vi "Mapping v10.5.2.vi"(5 "Simulate Spectra":bool, 7 "Simulate Drive":bool) -> ()   [LabVIEW 2010]
uses:
  ESA-C/TypeDefs/ESA-C Connection Settings.ctl
  TypeDefs/Mapping Spectra Params.ctl
  TypeDefs/Mapping Drive Params.ctl
  ESA-C/TypeDefs/ESA-C Set Positions.ctl
  ESA-C/TypeDefs/ESA-C Current Values.ctl
  iHR550/TypeDefs/iHR Current Values.ctl
  ITC503/TypeDefs/ITC503 Current Values.ctl
  TypeDefs/Mapping Input Parameters v10.5.1.ctl
  Symphony/TypeDefs/Symphony Area Format.ctl
  <vilib>/Utility/miscctls.llb/LVPointTypeDef.ctl
  Global Variables.vi
panel:
  in  "Input Parameters":T1={"Drive Connection Settings"={"Objective GPIB-Port"=4, "Stage GPIB-Port"=4, "Drive Selector"=0, "Drive Velocity (V/s)"=5.0}, "ITC503 Current Values"={"ITC503 Heater"=0.0, "ITC503 Temperature"=0.0, "ITC503 P"=0.0, "ITC503 I"=0.0, "ITC503 D"=0.0, "ITC503 Setpoint"=0.0, "ITC503 Gradient"=0.0, "ITC503 Heater Auto"=FALSE, "ITC503 PID Auto"=FALSE}, "Wavelengths (nm)"=[], "Drive Current Values"={"Voltages"={"Drive X Voltage"=0.0, "Drive Y Voltage"=0.0, "Drive Z Voltage"=0.0}, "Position"={"Drive X Position"=0.0, "Drive Y Position"=0.0, "Drive Z Position"=0.0}}, "iHR Current Values"={"iHR 550 Front Entrance"=0.0, "iHR550 Side Exit"=0.0, "iHR550 Wavelength"=897.9988, "iHR550 Exit Mirror"=2, "iHR550 Grating"="1", "Grating Index"=1}, "Spectra Settings"={"Integration Time"=1.0, "Repetitions"=1, "Mapping Spectra"=TRUE}, "CCD3500 Temperature"=0.0, "Simulate Drive"=FALSE, "Simulate Spectra"=FALSE, "JYCCDLib.IJYCCDReqd"=refnum, "CCD Area"={"XStart"=1, "YStart"=1, "XStop"=2048, "YStop"=512, "XBin"=1, "YBin"=1}, "CCD Gain"=1, "CCD ADC"=0} {"CCD ADC" items=["20 kHz       ", " 1 MHz       ", " 1 MHz Ultra ", "500 kHz Wrap"]; "CCD Gain" items=["High Light", "Best Dynamic Range", "High Sensitivity"]; "Drive Connection Settings"."Drive Velocity (V/s)" min=10.0 max=160.0 step=0.1 format="%.1f"; "Drive Connection Settings"."Drive Selector" items=["Obj.", "Stage"]; "Drive Connection Settings"."Stage GPIB-Port" min=1 max=20 step=1 format="%#.0f"; "Drive Connection Settings"."Objective GPIB-Port" min=1 max=20 step=1 format="%#.0f"; "ITC503 Current Values"."ITC503 Gradient" format="%.2f"; "ITC503 Current Values"."ITC503 Setpoint" min=-273.0 max=300000.0 step=0.0001 format="%.1f"; "ITC503 Current Values"."ITC503 I" format="%_1f"; "ITC503 Current Values"."ITC503 P" format="%_1f"; "ITC503 Current Values"."ITC503 Temperature" min=0.0 max=1645.0 step=1e-05 format="%.2f"; "ITC503 Current Values"."ITC503 Heater" min=0.0 max=100.0 step=0.01 scale=0.0..100.0; "Drive Current Values"."Position"."Drive Z Position" min=-273.0 max=300000.0 step=0.0001 format="%.1f"; "Drive Current Values"."Position"."Drive Y Position" min=-273.0 max=300000.0 step=0.0001 format="%.1f"; "Drive Current Values"."Position"."Drive X Position" min=-273.0 max=300000.0 step=0.0001 format="%.1f"; "Drive Current Values"."Voltages"."Drive Z Voltage" min=-273.0 max=300000.0 step=0.0001 format="%.1f"; "Drive Current Values"."Voltages"."Drive Y Voltage" min=-273.0 max=300000.0 step=0.0001 format="%.1f"; "Drive Current Values"."Voltages"."Drive X Voltage" min=-273.0 max=300000.0 step=0.0001 format="%.1f"; "iHR Current Values"."iHR550 Exit Mirror" items=["EntranceMirror", "ExitMirror", "Front", "Side"]; "Spectra Settings"."Repetitions" min=1 max=100 step=1; "Spectra Settings"."Integration Time" min=0.5 max=6000.0 step=1.0 format="%.1f"}
  out "JYCCDLib.IJYCCDReqd":refnum<k7>
  out "AutoClose":bool
  out "ITC503 Temperature":dbl caption="Sample (K)" min=10.0 max=160.0 step=0.1 format="%.3f"
  out "CCD3500 Temperature":dbl caption="CCD (°C)" min=10.0 max=160.0 step=0.1 format="%.1f"
  in  "CCD Current Rep.":string="0/0"
  in  "Pause":bool
  out "Current Position":T4 {"Position"."Drive Z Position" min=-273.0 max=300000.0 step=0.0001 format="%.1f"; "Position"."Drive Y Position" min=-273.0 max=300000.0 step=0.0001 format="%.1f"; "Position"."Drive X Position" min=-273.0 max=300000.0 step=0.0001 format="%.1f"; "Voltages"."Drive Z Voltage" min=-273.0 max=300000.0 step=0.0001 format="%.1f"; "Voltages"."Drive Y Voltage" min=-273.0 max=300000.0 step=0.0001 format="%.1f"; "Voltages"."Drive X Voltage" min=-273.0 max=300000.0 step=0.0001 format="%.1f"}
  out "Target Position":T8={"Drive X Set"=10.0, "Drive Y Set"=10.0, "Drive Z Set"=10.0} {"Drive X Set" min=10.0 max=160.0 step=0.1 format="%.1f"; "Drive Z Set" min=10.0 max=160.0 step=0.1 format="%.1f"; "Drive Y Set" min=10.0 max=160.0 step=0.1 format="%.1f"}
  out "Progress":u8(slide) max=10 scale=0.0..100.0
  out "Objective Running":bool caption="Obj."
  out "CCD Running":bool caption="CCD"
  in  "Save Map":bool
  in  "Spectra Params":T6={"Integration Time"=10.0, "Repetitions"=10, "Mapping Spectra"=TRUE} {"Repetitions" min=1 max=100 step=1; "Integration Time" min=0.5 max=6000.0 step=1.0 format="%.1f"}
  in  "Drive Settings":T2={"Objective GPIB-Port"=4, "Stage GPIB-Port"=4, "Drive Selector"=0, "Drive Velocity (V/s)"=5.0} {"Drive Velocity (V/s)" min=10.0 max=160.0 step=0.1 format="%.1f"; "Drive Selector" items=["Obj.", "Stage"]; "Stage GPIB-Port" min=1 max=20 step=1 format="%#.0f"; "Objective GPIB-Port" min=1 max=20 step=1 format="%#.0f"}
  in  "Z Position":dbl caption="Z (µm)" min=0.0 max=100.0 step=0.1 format="%.1f"
  in  "Mapping Params":T9={"X Start Position"=0.0, "X Stop Position"=10.0, "Y Start Position"=0.0, "Y Stop Position"=10.0, "Step Size"=1.0} {"Step Size" min=0.1 max=30.0 step=0.1 format="%.1f"; "Y Stop Position" min=0.0 max=30.0 step=0.1 format="%.1f"; "Y Start Position" min=0.0 max=30.0 step=0.1 format="%.1f"; "X Stop Position" min=0.0 max=30.0 step=0.1 format="%.1f"; "X Start Position" min=0.0 max=30.0 step=0.1 format="%.1f"}
  in  "Exit":bool
  out "Measuring":bool
  in  "Start":bool
  out "Filename":string
  out "Full Data":dbl[][](array[numeric])
  out "Live Data":dbl[][](array[numeric])
  in  "ITC503 Current Values":T3 {"ITC503 Gradient" format="%.2f"; "ITC503 Setpoint" min=-273.0 max=300000.0 step=0.0001 format="%.1f"; "ITC503 I" format="%_1f"; "ITC503 P" format="%_1f"; "ITC503 Temperature" min=0.0 max=1645.0 step=1e-05 format="%.2f"; "ITC503 Heater" min=0.0 max=100.0 step=0.01 scale=0.0..100.0}
  in  "iHR Current Values":T5={"iHR 550 Front Entrance"=0.0, "iHR550 Side Exit"=0.0, "iHR550 Wavelength"=897.9988, "iHR550 Exit Mirror"=2, "iHR550 Grating"="1", "Grating Index"=1} {"iHR550 Exit Mirror" items=["EntranceMirror", "ExitMirror", "Front", "Side"]}
  in  "Wavelengths (nm)":dbl[](array[numeric])
  # "Status"
  # "Active"
  # "Target"
  # "Current"
  # "Parameters"
  # "Spectral"
  # "Spectral / Video Mapping"
  # "Mapping"
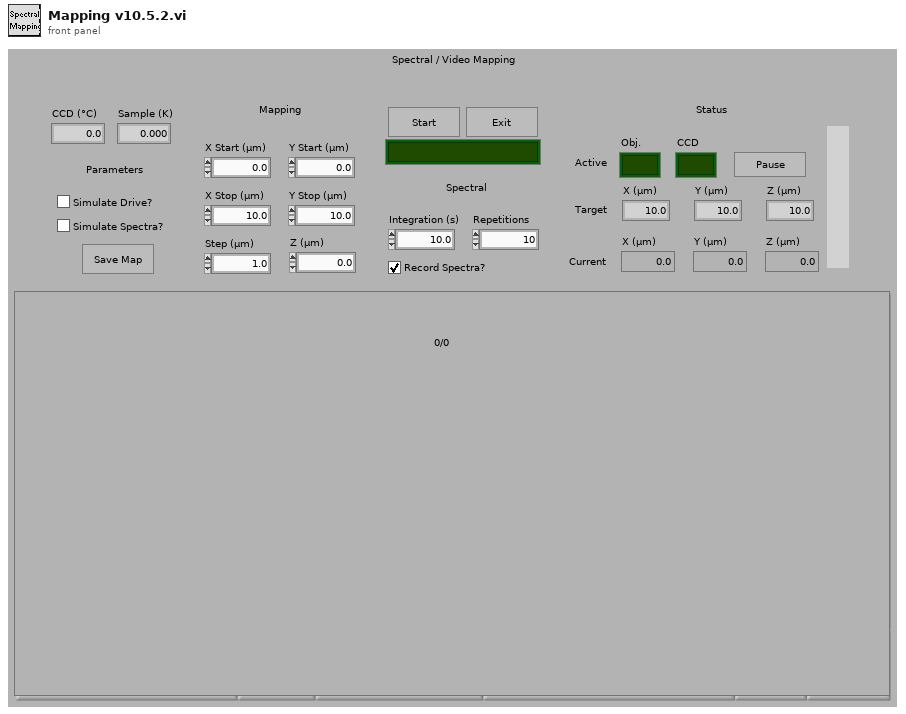
[diagram p1: front panel]
types:
  T1 = typedef "Mapping Input Parameters v10.5.1.ctl" = cluster{"Drive Connection Settings":T2, "ITC503 Current Values":T3, "Wavelengths (nm)":dbl[], "Drive Current Values":T4, "iHR Current Values":T5, "Spectra Settings":T6, "CCD3500 Temperature":dbl, "Simulate Drive":bool, "Simulate Spectra":bool, "JYCCDLib.IJYCCDReqd":refnum<k7>, "CCD Area":T7, "CCD Gain":u16, "CCD ADC":u16}
  T2 = typedef "ESA-C Connection Settings.ctl" = cluster{"Objective GPIB-Port":i32, "Stage GPIB-Port":i32, "Drive Selector":u16, "Drive Velocity (V/s)":dbl}
  T3 = typedef "ITC503 Current Values.ctl" = cluster{"ITC503 Heater":dbl, "ITC503 Temperature":dbl, "ITC503 P":dbl, "ITC503 I":dbl, "ITC503 D":dbl, "ITC503 Setpoint":dbl, "ITC503 Gradient":dbl, "ITC503 Heater Auto":bool, "ITC503 PID Auto":bool}
  T4 = typedef "ESA-C Current Values.ctl" = cluster{"Voltages":cluster{"Drive X Voltage":dbl, "Drive Y Voltage":dbl, "Drive Z Voltage":dbl}, "Position":cluster{"Drive X Position":dbl, "Drive Y Position":dbl, "Drive Z Position":dbl}}
  T5 = typedef "iHR Current Values.ctl" = cluster{"iHR 550 Front Entrance":dbl, "iHR550 Side Exit":dbl, "iHR550 Wavelength":dbl, "iHR550 Exit Mirror":i32, "iHR550 Grating":string, "Grating Index":i32}
  T6 = typedef "Mapping Spectra Params.ctl" = cluster{"Integration Time":dbl, "Repetitions":u16, "Mapping Spectra":bool}
  T7 = typedef "Symphony Area Format.ctl" = cluster{"XStart":i32, "YStart":i32, "XStop":i32, "YStop":i32, "XBin":i32, "YBin":i32}
  T8 = typedef "ESA-C Set Positions.ctl" = cluster{"Drive X Set":dbl, "Drive Y Set":dbl, "Drive Z Set":dbl}
  T9 = typedef "Mapping Drive Params.ctl" = cluster{"X Start Position":dbl, "X Stop Position":dbl, "Y Start Position":dbl, "Y Stop Position":dbl, "Step Size":dbl}
  T10 = typedef "LVPointTypeDef.ctl" = cluster{"Horizontal":i16, "Vertical":i16}
  T11 = cluster{"Drive X Position":dbl, "Drive Y Position":dbl, "Drive Z Position":dbl}
  T12 = typedef "NPC3SG Set Positions.ctl" = cluster{"Drive X Set":dbl, "Drive Y Set":dbl, "Drive Z Set":dbl}
  T13 = cluster{"Intensities":dbl[], "Wavelengths":dbl[]}[]
  T14 = cluster{"Intensities":dbl[], "Wavelengths":dbl[]}
  T15 = enum32{"invalid app kind", "Development System", "Run Time System", "Student Edition", "Embedded LabVIEW", "Evaluation", "Custom"}
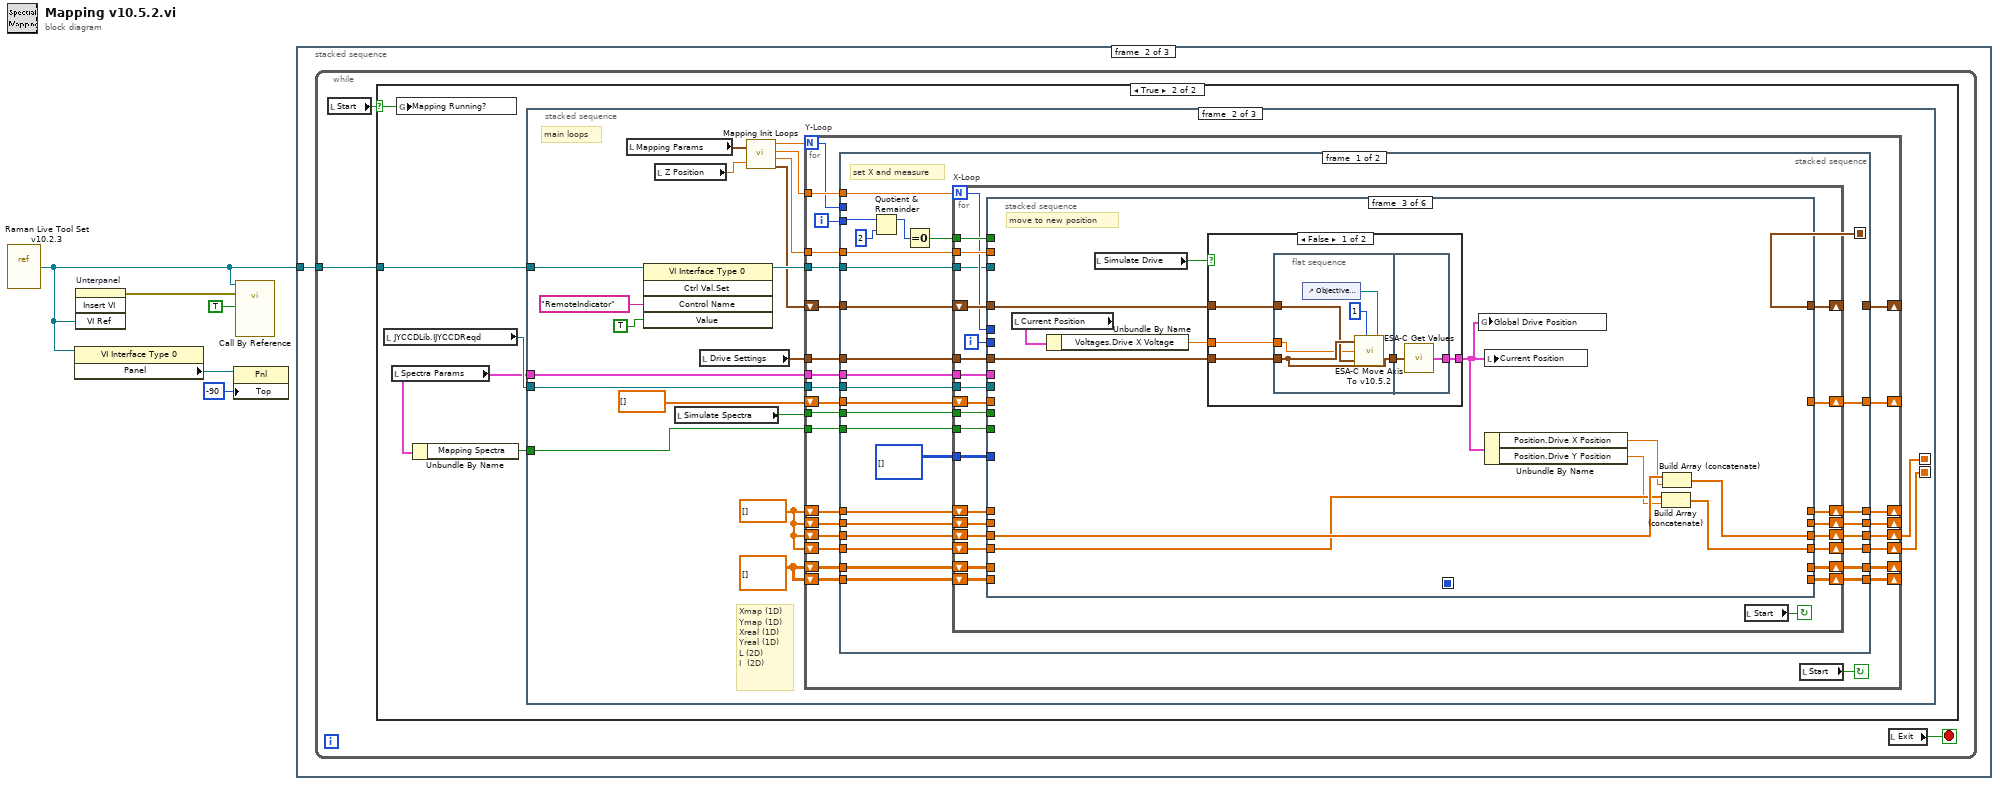
[diagram p0: block diagram]
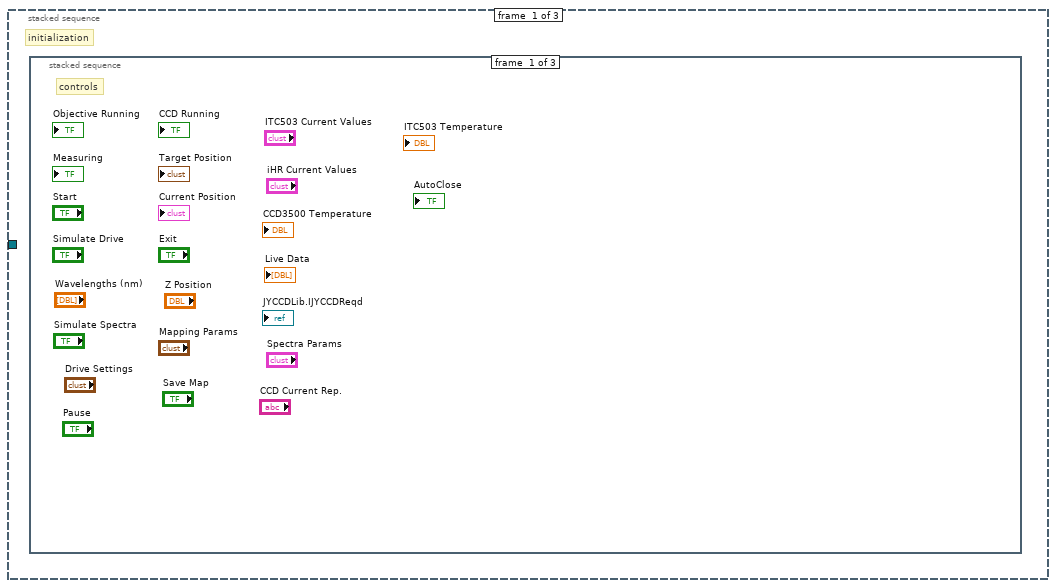
[diagram p2: hidden frame]
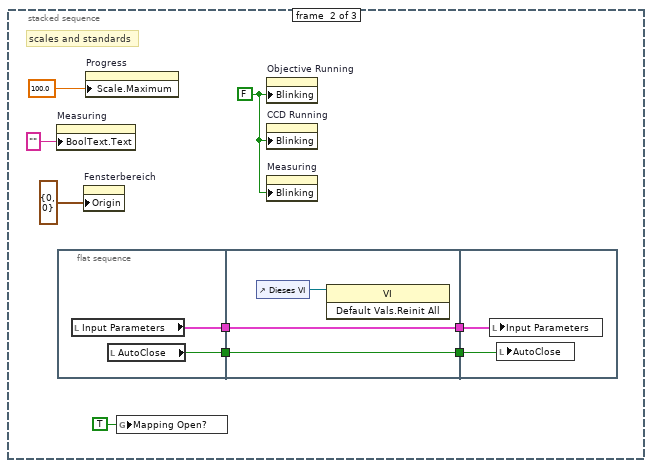
[diagram p3: hidden frame]
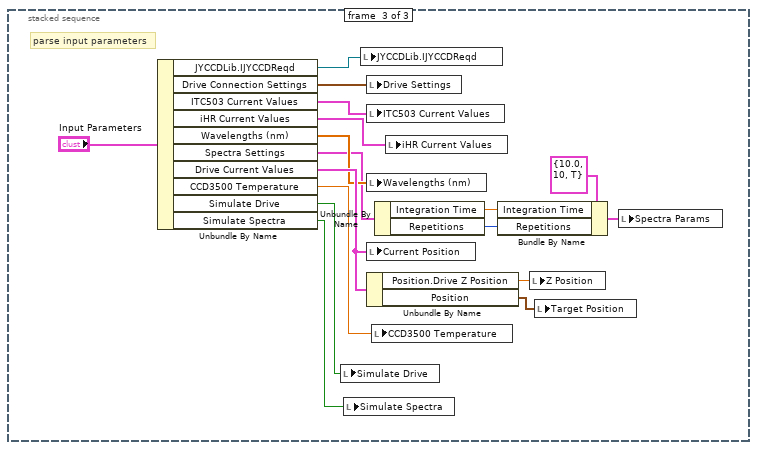
[diagram p4: hidden frame]
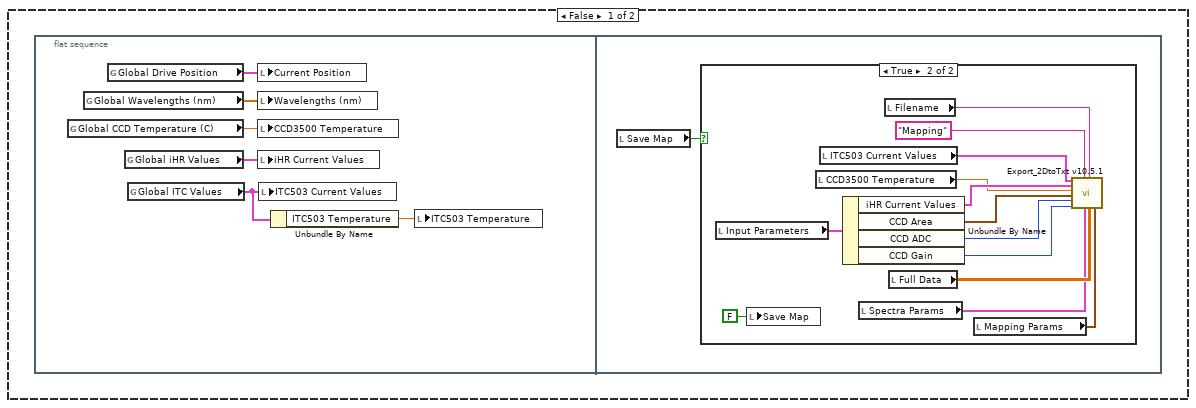
[diagram p5: hidden frame]
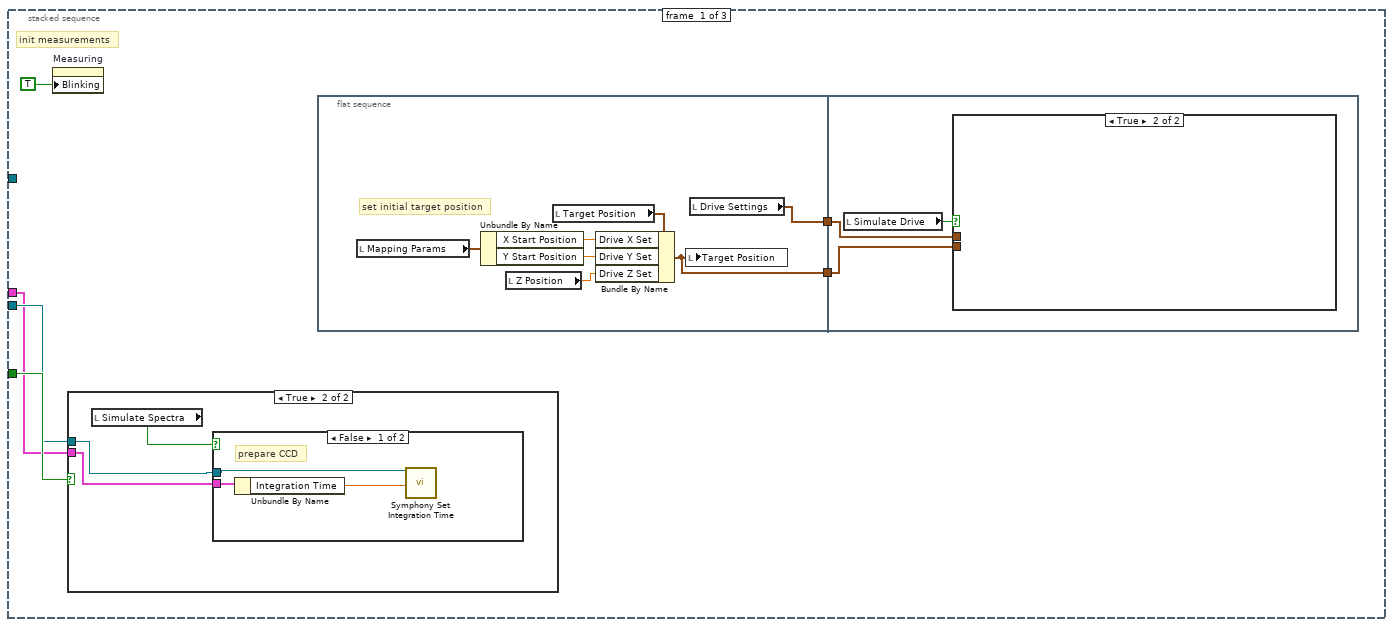
[diagram p7: hidden frame]
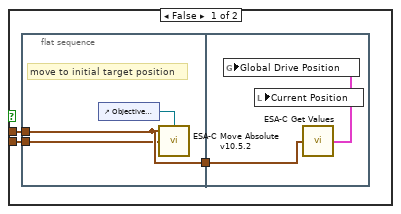
[diagram p8: hidden frame]
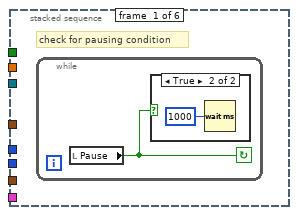
[diagram p11: hidden frame]
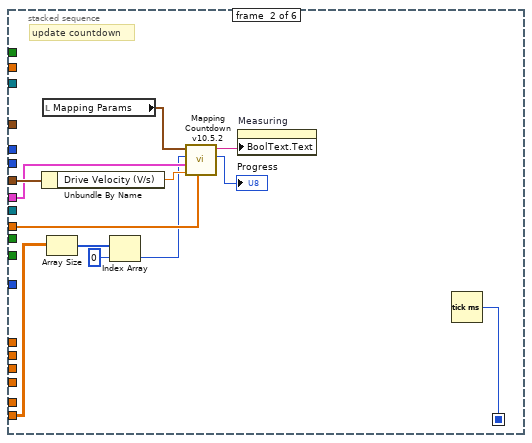
[diagram p13: hidden frame]
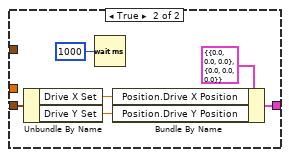
[diagram p14: hidden frame]
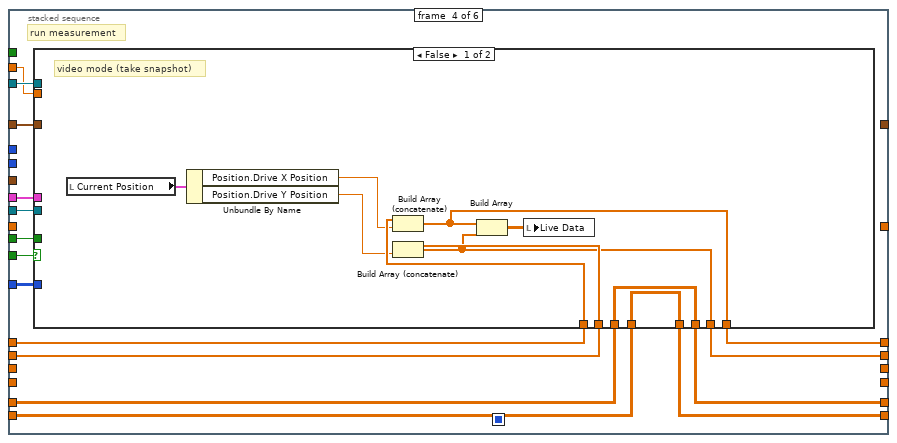
[diagram p15: hidden frame]
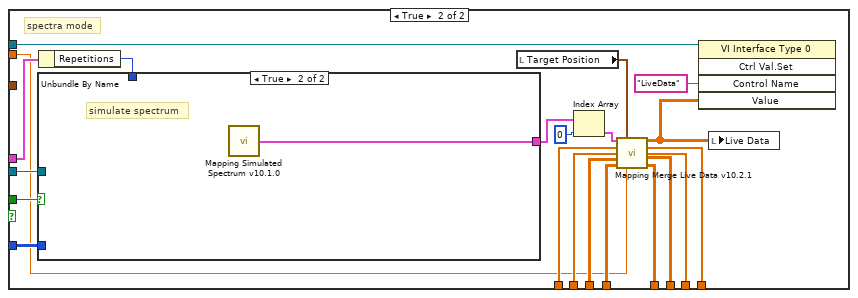
[diagram p16: hidden frame]
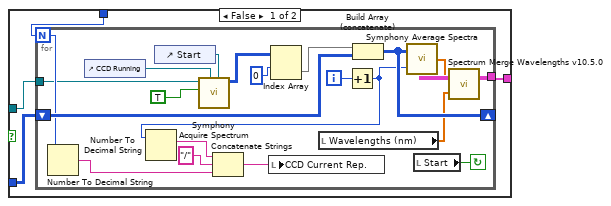
[diagram p17: hidden frame]
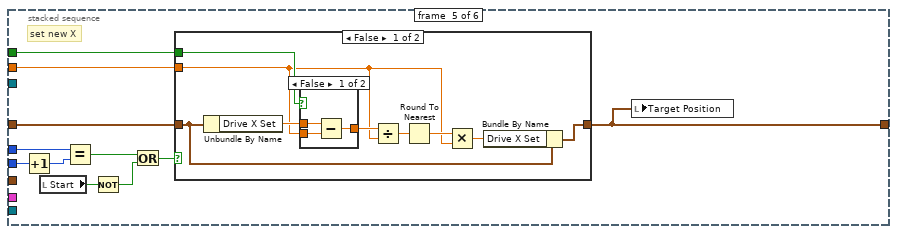
[diagram p18: hidden frame]
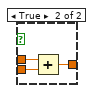
[diagram p19: hidden frame]
diagram:
  n1 = vi-ref "Raman Live Tool Set v10.2.3.vi"() -> (w3:refnum<vi>)
  n2 = property class="VI Interface Type 0"(reference=w3) -> ("Panel"=w2:refnum<vi>)  [unwired: 1 in, 2 out]
  n3 = invoke on="Unterpanel" class="Unterpanel" method="Insert VI"("VI Ref"=w3) -> (error out=w5:errorcluster)  [unwired: 3 in, 3 out]
  n4 = property class="Pnl"(reference=w2, "Top"=-90 ("Position:Oben")) -> ()  [unwired: 1 in, 2 out]
  n5 = call-by-ref "?"(reference=w3, error in=w5, "RemoteIndicator"=TRUE) -> ()  [unwired: 3 in, 2 out]
  n6 = stacked-sequence {
    tunnel: w3 -> [_ w39 w412]
    frame #0 {
      # "initialization"
      n7 = stacked-sequence {
        frame #0 {
          # "controls"
        }
        frame #1 {
          w12 = FALSE ("Blinkend")
          # "scales and standards"
          n8 = property on="Measuring" class="Bool (strict)"("BoolText.Text"="" ("Boolescher Text.Text")) -> ()  [unwired: 2 in, 2 out]
          n9 = flat-sequence {
            tunnel: [w16] -> w9
            tunnel: [w15] -> w6
            tunnel: [w18] -> w10
            tunnel: w9 -> [w18]
            tunnel: [w17] -> w7
            tunnel: w6 -> [w17]
            tunnel: w10 -> [w21]
            tunnel: w7 -> [w20]
            frame #0 {
              n10 = local read "Input Parameters"() -> (w16:T1)
              n11 = local read "AutoClose"() -> (w15:bool)
            }
            frame #1 {
              n12 = control-ref of="Dieses VI"() -> (w19:refnum<vi>)
              n13 = invoke class="VI" method="Default Vals.Reinit All"(reference=w19) -> ()  [unwired: 2 in, 3 out]
            }
            frame #2 {
              n14 = local write "Input Parameters"(w21) -> ()
              n15 = local write "AutoClose"(w20) -> ()
            }
          }
          n16 = property on="Fensterbereich" class="Pane"("Origin"=T10 {"Horizontal"=0, "Vertical"=0}) -> ()  [unwired: 2 in, 2 out]
          n17 = property on="Progress" class="Slide (strict)"("Scale.Maximum"=100.0 ("Skalierung.Bereich:Maximum")) -> ()  [unwired: 2 in, 2 out]
          n18 = global write "Global Variables.vi" "Mapping Open?"(TRUE ("Mapping Open?")) -> ()
          n19 = property on="Objective Running" class="Bool (strict)"("Blinking"=w12) -> ()  [unwired: 2 in, 2 out]
          n20 = property on="CCD Running" class="Bool (strict)"("Blinking"=w12) -> ()  [unwired: 2 in, 2 out]
          n21 = property on="Measuring" class="Bool (strict)"("Blinking"=w12) -> ()  [unwired: 2 in, 2 out]
        }
        frame #2 {
          # "parse input parameters"
          n22 = Unbundle By Name("Input Parameters") -> ("JYCCDLib.IJYCCDReqd"=w24:refnum<k7>, "Drive Connection Settings"=w36:T2, "ITC503 Current Values"=w37:T3, "iHR Current Values"=w27:T5, "Wavelengths (nm)"=w35:dbl[], "Spectra Settings"=w33:T6, "Drive Current Values"=w38:T4, "CCD3500 Temperature"=w28:dbl, "Simulate Drive"=w26:bool, "Simulate Spectra"=w25:bool)
          n23 = local write "Simulate Drive"(w26) -> ()
          n24 = local write "Simulate Spectra"(w25) -> ()
          n25 = local write "JYCCDLib.IJYCCDReqd"(w24) -> ()
          n26 = local write "Drive Settings"(w36) -> ()
          n27 = local write "ITC503 Current Values"(w37) -> ()
          n28 = local write "Wavelengths (nm)"(w35) -> ()
          n29 = local write "Current Position"(w38) -> ()
          n30 = Unbundle By Name(w38) -> ("Position.Drive Z Position"=w34:dbl, "Position"=w23:T11)
          n31 = local write "CCD3500 Temperature"(w28) -> ()
          n32 = Unbundle By Name(w33) -> ("Integration Time"=w31:dbl, "Repetitions"=w30:u16)
          n33 = local write "iHR Current Values"(w27) -> ()
          n34 = Bundle By Name(cluster=T6 {"Integration Time"=10.0, "Repetitions"=10, "Mapping Spectra"=TRUE} ("Mapping Spectra Settings"), "Integration Time"=w31, "Repetitions"=w30) -> (w29:T6)
          n35 = local write "Z Position"(w34) -> ()
          n36 = local write "Target Position"(w23) -> ()
          n37 = local write "Spectra Params"(w29) -> ()
        }
      }
    }
    frame #1 {
      n38 = while {
        tunnel: w39 -> [w42]
        stop <- w41 stop-if-true
        n39 = local read "Start"() -> (w40:bool)
        n40 = case shown="True" w40 {
          selector: w40 -> [_ w63]
          tunnel: w42 -> [_ w67]
          frame False {
            n41 = flat-sequence {
              frame #0 {
                n42 = global read "Global Variables.vi" "Global CCD Temperature (C)"() -> (w48:dbl)
                n43 = global read "Global Variables.vi" "Global Wavelengths (nm)"() -> (w46:dbl[])
                n44 = global read "Global Variables.vi" "Global Drive Position"() -> (w47:T4)
                n45 = global read "Global Variables.vi" "Global iHR Values"() -> (w45:T5)
                n46 = global read "Global Variables.vi" "Global ITC Values"() -> (w44:T3)
                n47 = local write "Current Position"(w47) -> ()
                n48 = local write "Wavelengths (nm)"(w46) -> ()
                n49 = local write "CCD3500 Temperature"(w48) -> ()
                n50 = local write "iHR Current Values"(w45) -> ()
                n51 = local write "ITC503 Current Values"(w44) -> ()
                n52 = Unbundle By Name(w44) -> ("ITC503 Temperature"=w43:dbl)
                n53 = local write "ITC503 Temperature"(w43) -> ()
              }
              frame #1 {
                n54 = local read "Save Map"() -> (w49:bool)
                n55 = case shown="True" w49 {
                  frame False {
                  }
                  frame True {
                    n56 = local read "Input Parameters"() -> (w58:T1)
                    n57 = local write "Save Map"(FALSE ("Save Map")) -> ()
                    n58 = local read "CCD3500 Temperature"() -> (w52:dbl)
                    n59 = local read "ITC503 Current Values"() -> (w55:T3)
                    n60 = Unbundle By Name(w58) -> ("iHR Current Values"=w53:T5, "CCD Area"=w54:T7, "CCD ADC"=w57:u16, "CCD Gain"=w56:u16)
                    n61 = local read "Spectra Params"() -> (w51:T6)
                    n62 = local read "Filename"() -> (w61:string)
                    n63 = local read "Full Data"() -> (w59:dbl[][])
                    n64 = local read "Mapping Params"() -> (w50:T9)
                    n65 = call "Export_2DtoTxt v10.5.1.vi"("ITC503 Current Values"=w55, "iHR Current Values"=w53, "CCD Temperature"=w52, "CCD Area"=w54, "CCD ADC"=w57, "CCD Gain"=w56, "Export Type"="Mapping", "Spectra Settings"=w51, "Filename"=w61, "Data (2D)"=w59, "Mapping Parameters"=w50) -> ()  [unwired: 8 in, 1 out]
                  }
                }
              }
            }
          }
          frame True {
            n66 = local read "JYCCDLib.IJYCCDReqd"() -> (w65:refnum<k7>)
            n67 = local read "Spectra Params"() -> (w64:T6)
            n68 = global write "Global Variables.vi" "Mapping Running?"(w63) -> ()
            n69 = Unbundle By Name(w64) -> ("Mapping Spectra"=w66:bool)
            n70 = stacked-sequence {
              seq-local: [_ w98 _] -> [_ _ w387]
              seq-local: [_ w99 _] -> [_ _ w386]
              tunnel: w67 -> [_ w109 _]
              tunnel: w66 -> [w72 w108 w388]
              tunnel: w64 -> [w70 w106 _]
              tunnel: w65 -> [w71 w105 _]
              frame #0 {
                # "init measurements"
                n71 = property on="Measuring" class="Bool (strict)"("Blinking"=TRUE ("Blinkend")) -> ()  [unwired: 2 in, 2 out]
                n72 = case shown="True" w72 {
                  tunnel: w71 -> [_ w94]
                  tunnel: w70 -> [_ w93]
                  frame False {
                  }
                  frame True {
                    n73 = local read "Simulate Spectra"() -> (w92:bool)
                    n74 = case shown="False" w92 {
                      tunnel: w94 -> [w97 _]
                      tunnel: w93 -> [w96 _]
                      frame False {
                        # "prepare CCD"
                        n75 = Unbundle By Name(w96) -> ("Integration Time"=w95:dbl)
                        n76 = call "Symphony Set Integration Time.vi"("JYCCDLib.IJYCCDReqd"=w97, "Integration (s)"=w95) -> ()  [unwired: 13 in, 1 out]
                      }
                      frame True {
                      }
                    }
                  }
                }
                n77 = flat-sequence {
                  tunnel: [w75] -> w69
                  tunnel: [w74] -> w68
                  tunnel: w69 -> [w81]
                  tunnel: w68 -> [w82]
                  frame #0 {
                    # "set initial target position"
                    n78 = local read "Mapping Params"() -> (w80:T9)
                    n79 = Unbundle By Name(w80) -> ("X Start Position"=w78:dbl, "Y Start Position"=w77:dbl)
                    n80 = local read "Z Position"() -> (w76:dbl)
                    n81 = local read "Target Position"() -> (w79:T8)
                    n82 = Bundle By Name(cluster=w79, "Drive X Set"=w78, "Drive Y Set"=w77, "Drive Z Set"=w76) -> (w75:T8)
                    n83 = local write "Target Position"(w75) -> ()
                    n84 = local read "Drive Settings"() -> (w74:T2)
                  }
                  frame #1 {
                    n85 = local read "Simulate Drive"() -> (w83:bool)
                    n86 = case shown="True" w83 {
                      tunnel: w82 -> [w86 _]
                      tunnel: w81 -> [w84 _]
                      frame False {
                        n87 = flat-sequence {
                          tunnel: w86 -> [w88]
                          tunnel: [w88] -> w85
                          tunnel: w84 -> [w87]
                          tunnel: w85 -> [w91]
                          frame #0 {
                            # "move to initial target position"
                            n88 = control-ref of="Objective Running"() -> (w89:refnum<vi>)
                            n89 = call "ESA-C Move Absolute v10.5.2.vi"("Running"=w89, "Drive New Abs. Positions"=w87, "Drive Connection Settings"=w88) -> ()  [unwired: 2 in]
                          }
                          frame #1 {
                            n90 = call "ESA-C Get Values.vi"("Drive Connection Settings"=w91) -> ("Drive Current Values"=w90:T4)
                            n91 = global write "Global Variables.vi" "Global Drive Position"(w90) -> ()
                            n92 = local write "Current Position"(w90) -> ()
                          }
                        }
                      }
                      frame True {
                      }
                    }
                  }
                }
              }
              frame #1 {
                w117 = dbl[][] []
                w100 = dbl[] []
                # "main loops"
                # "Xmap (1D)\nYmap (1D)\nXreal (1D)\nYreal (1D)\nL (2D)\nI  (2D)"
                n93 = local read "Mapping Params"() -> (w103:T9)
                n94 = invoke class="VI Interface Type 0" method="Ctrl Val.Set"(reference=w109, "Control Name"="RemoteIndicator" ("Elementname"), "Value"=TRUE) -> (reference out=w111:refnum<vi>)  [unwired: 2 in, 4 out]
                n95 = local read "Z Position"() -> (w102:dbl)
                n96 = local read "Simulate Spectra"() -> (w101:bool)
                n97 = local read "Drive Settings"() -> (w104:T2)
                n98 = call "Mapping Init Loops.vi"("Z Position"=w102, "Mapping Params"=w103) -> ("Start Positions"=w110:T12, "Step Size"=w112:dbl, "X Steps"=w113:dbl, "Y Steps"=w114:dbl)
                n99 = for "Y-Loop" {
                  N: w114 -> [w130]
                  tunnel: w113 -> [w143]
                  tunnel: w112 -> [w142]
                  shift-right: [w128] -> _
                  shift-left: w110 -> [w129]
                  shift-right: [w134] -> _
                  shift-left: w117 -> [w138]
                  shift-right: [w135] -> _
                  shift-left: w117 -> [w139]
                  shift-right: [w137] -> _
                  shift-left: w100 -> [w141]
                  shift-right: [w136] -> _
                  shift-left: w100 -> [w140]
                  tunnel: w111 -> [w132]
                  tunnel: w101 -> [w131]
                  tunnel: w104 -> [w127]
                  tunnel: w108 -> [w126]
                  tunnel: w106 -> [w125]
                  shift-right: [w123] -> _
                  shift-left: dbl[] [] -> [w124]
                  tunnel: w105 -> [w122]
                  shift-right: [w119] -> w99
                  shift-left: w100 -> [w120]
                  shift-right: [w118] -> w98
                  shift-left: w100 -> [w121]
                  i -> [w133]
                  stop <- w144 continue-if-true
                  n100 = stacked-sequence {
                    seq-local: [w158 _] -> [_ w359]
                    tunnel: w143 -> [w173 _]
                    tunnel: w142 -> [w172 w360]
                    tunnel: w141 -> [w171 _]
                    tunnel: w140 -> [w170 _]
                    tunnel: w139 -> [w169 _]
                    tunnel: w138 -> [w145 _]
                    tunnel: [w168 _] -> w137
                    tunnel: [w167 _] -> w136
                    tunnel: [w166 _] -> w135
                    tunnel: [w165 _] -> w134
                    tunnel: w133 -> [w162 w363]
                    tunnel: w132 -> [w160 _]
                    tunnel: w131 -> [w159 _]
                    tunnel: w130 -> [_ w361]
                    tunnel: w129 -> [w157 _]
                    tunnel: [_ w357] -> w128
                    tunnel: w127 -> [w156 w358]
                    tunnel: w126 -> [w155 _]
                    tunnel: w125 -> [w154 _]
                    tunnel: w124 -> [w153 _]
                    tunnel: [w152 _] -> w123
                    tunnel: w122 -> [w151 _]
                    tunnel: w121 -> [w149 _]
                    tunnel: w120 -> [w148 _]
                    tunnel: [w147 _] -> w119
                    tunnel: [w146 _] -> w118
                    frame #0 {
                      # "set X and measure"
                      n101 = Quotient & Remainder(x=w162, y=2) -> (x-y*floor(x/y)=w163:i32)  [unwired: 1 out]
                      n102 = Equal To 0?(x=w163) -> (x = 0?=w161:bool)
                      n103 = for "X-Loop" {
                        N: w173 -> [w187]
                        tunnel: w172 -> [w199]
                        shift-right: [w198] -> w158
                        shift-left: w157 -> [w200]
                        shift-right: [w193] -> w168
                        shift-left: w171 -> [w197]
                        shift-right: [w192] -> w167
                        shift-left: w170 -> [w196]
                        shift-right: [w190] -> w166
                        shift-left: w169 -> [w195]
                        shift-right: [w191] -> w165
                        shift-left: w145 -> [w194]
                        tunnel: w161 -> [w189]
                        tunnel: w160 -> [w186]
                        tunnel: w159 -> [w185]
                        tunnel: w156 -> [w184]
                        tunnel: w155 -> [w183]
                        tunnel: w154 -> [w182]
                        shift-right: [w181] -> w152
                        shift-left: w153 -> [w180]
                        tunnel: w151 -> [w179]
                        tunnel: u16[][] [] -> [w178]
                        shift-right: [w174] -> w146
                        shift-left: w149 -> [w177]
                        shift-right: [w175] -> w147
                        shift-left: w148 -> [w176]
                        i -> [w188]
                        stop <- w201 continue-if-true
                        n104 = stacked-sequence {
                          seq-local: [_ w208 _ _ _ _] -> [_ _ _ _ _ w348]
                          tunnel: w200 -> [_ _ w227 w261 w325 _]
                          tunnel: w199 -> [_ _ _ w246 w323 _]
                          tunnel: [_ _ _ _ w322 _] -> w198
                          tunnel: w197 -> [_ _ _ w260 _ _]
                          tunnel: w196 -> [_ _ _ w259 _ _]
                          tunnel: w195 -> [_ _ _ w257 _ _]
                          tunnel: w194 -> [_ w207 _ w258 _ _]
                          tunnel: [_ _ _ w256 _ _] -> w193
                          tunnel: [_ _ _ w255 _ _] -> w192
                          tunnel: [_ _ _ w254 _ _] -> w191
                          tunnel: [_ _ _ w253 _ _] -> w190
                          tunnel: w189 -> [_ _ _ _ w324 _]
                          tunnel: w188 -> [_ _ _ _ w328 _]
                          tunnel: w187 -> [_ _ _ _ w326 _]
                          tunnel: w186 -> [_ _ _ w252 _ _]
                          tunnel: w185 -> [_ _ _ w251 _ _]
                          tunnel: w184 -> [_ w211 w225 _ _ _]
                          tunnel: w183 -> [_ _ _ w250 _ _]
                          tunnel: w182 -> [_ w210 _ w248 _ _]
                          tunnel: [_ _ _ _ _ w345] -> w181
                          tunnel: w180 -> [_ w209 _ _ _ w347]
                          tunnel: w179 -> [_ _ _ w249 _ _]
                          tunnel: w178 -> [_ _ _ w247 _ _]
                          tunnel: w177 -> [_ _ w222 _ _ _]
                          tunnel: w176 -> [_ _ w221 _ _ _]
                          tunnel: [_ _ w218 _ _ _] -> w175
                          tunnel: [_ _ w217 _ _ _] -> w174
                          frame #0 {
                            # "check for pausing condition"
                            n105 = while {
                              stop <- w202 continue-if-true
                              n106 = local read "Pause"() -> (w202:bool)
                              n107 = case shown="True" w202 {
                                frame False {
                                }
                                frame True {
                                n108 = Wait (ms)(milliseconds to wait=u32 1000) -> ()  [unwired: 1 out]
                                }
                              }
                            }
                          }
                          frame #1 {
                            # "update countdown"
                            n109 = Unbundle By Name(w211) -> ("Drive Velocity (V/s)"=w212:dbl)
                            n110 = local read "Mapping Params"() -> (w215:T9)
                            n111 = Array Size(array=w207) -> (size(s)=w206:i32[])
                            n112 = Index Array(array=w206, index=0) -> (element=w204:i32)
                            n113 = call "Mapping Countdown v10.5.2.vi"("Execution Times (s)"=w209, "Drive Velocity"=w212, "Mapping Spectra Settings"=w210, "Ready Steps"=w204, "Mapping Drive Parameters"=w215) -> ("Progress"=→"Progress":i16, "Time String"=w213:string)  [unwired: 5 in]
                            n114 = property on="Measuring" class="Bool (strict)"("BoolText.Text"=w213) -> ()  [unwired: 2 in, 2 out]
                            n115 = Tick Count (ms)() -> (millisecond timer value=w208:u32)
                          }
                          frame #2 {
                            # "move to new position"
                            n116 = local read "Current Position"() -> (w224:T4)
                            n117 = Unbundle By Name(w224) -> ("Voltages.Drive X Voltage"=w223:dbl)
                            n118 = local read "Simulate Drive"() -> (w226:bool)
                            n119 = case shown="False" w226 {
                              tunnel: w227 -> [w231 w244]
                              tunnel: [w230 w241] -> w216
                              tunnel: w225 -> [w229 _]
                              tunnel: w223 -> [w228 _]
                              frame False {
                                n120 = flat-sequence {
                                tunnel: w231 -> [w236]
                                tunnel: [w237] -> w232
                                tunnel: w229 -> [w237]
                                tunnel: w228 -> [w233]
                                tunnel: w232 -> [w239]
                                tunnel: [w238] -> w230
                                frame #0 {
                                n121 = control-ref of="Objective Running"() -> (w234:refnum<vi>)
                                n122 = call "ESA-C Move Axis To v10.5.2.vi"("Drive Connection Settings"=w237, "Axis"=1, "Current Voltage (V)"=w233, "Drive New Abs. Positions"=w236, "Running"=w234) -> ()  [unwired: 2 in]
                                }
                                frame #1 {
                                n123 = call "ESA-C Get Values.vi"("Drive Connection Settings"=w239) -> ("Drive Current Values"=w238:T4)
                                }
                                }
                              }
                              frame True {
                                n124 = Unbundle By Name(w244) -> ("Drive X Set"=w245:dbl, "Drive Y Set"=w242:dbl)
                                n125 = Wait (ms)(milliseconds to wait=u32 1000 ("Zu wartende ms")) -> ()  [unwired: 1 out]
                                n126 = Bundle By Name(cluster=T4 {"Voltages"={"Drive X Voltage"=0.0, "Drive Y Voltage"=0.0, "Drive Z Voltage"=0.0}, "Position"={"Drive X Position"=0.0, "Drive Y Position"=0.0, "Drive Z Position"=0.0}} ("Drive Current Values"), "Position.Drive X Position"=w245, "Position.Drive Y Position"=w242) -> (w241:T4)
                              }
                            }
                            n127 = global write "Global Variables.vi" "Global Drive Position"(w216) -> ()
                            n128 = local write "Current Position"(w216) -> ()
                            n129 = Unbundle By Name(w216) -> ("Position.Drive X Position"=w220:dbl, "Position.Drive Y Position"=w219:dbl)
                            n130 = Build Array (concatenate)(w221, w219) -> (w218:dbl[])
                            n131 = Build Array (concatenate)(w222, w220) -> (w217:dbl[])
                          }
                          frame #3 {
                            # "run measurement"
                            n132 = case shown="False" w250 {
                              tunnel: w261 -> [_ _]
                              tunnel: w260 -> [w268 w289]
                              tunnel: w259 -> [w267 w288]
                              tunnel: w258 -> [w270 w286]
                              tunnel: w257 -> [w271 w287]
                              tunnel: [w265 w283] -> w256
                              tunnel: [w266 w282] -> w255
                              tunnel: [w270 w285] -> w254
                              tunnel: [w271 w284] -> w253
                              tunnel: w252 -> [_ w291]
                              tunnel: w251 -> [_ w290]
                              tunnel: w249 -> [_ w279]
                              tunnel: w248 -> [_ w278]
                              tunnel: w247 -> [_ w276]
                              tunnel: w246 -> [_ w272]
                              frame False {
                                # "video mode (take snapshot)"
                                n133 = local read "Current Position"() -> (w269:T4)
                                n134 = Unbundle By Name(w269) -> ("Position.Drive X Position"=w264:dbl, "Position.Drive Y Position"=w263:dbl)
                                n135 = Build Array (concatenate)(w268, w264) -> (w265:dbl[])
                                n136 = Build Array (concatenate)(w267, w263) -> (w266:dbl[])
                                n137 = Build Array(w265, w266) -> (w262:dbl[][])
                                n138 = local write "Live Data"(w262) -> ()
                              }
                              frame True {
                                # "spectra mode"
                                n139 = Unbundle By Name(w278) -> ("Repetitions"=w277:u16)
                                n140 = case shown="True" w290 {
                                tunnel: [w295 w317] -> w275
                                tunnel: w279 -> [w296 _]
                                tunnel: w277 -> [w294 _]
                                tunnel: w276 -> [w293 _]
                                frame False {
                                n141 = for {
                                N: w294 -> [w303]
                                shift-right: [w314] -> _
                                shift-left: w293 -> [w315]
                                tunnel: [w312] -> w295
                                tunnel: w296 -> [w301]
                                i -> [w316]
                                stop <- w310 continue-if-true
                                n142 = Number To Decimal String(number=w303) -> (decimal integer string=w306:string)  [unwired: 1 in]
                                n143 = control-ref of="CCD Running"() -> (w309:refnum<vi>)
                                n144 = control-ref of="Start"() -> (w308:refnum<vi>)
                                n145 = call "Symphony Acquire Spectrum.vi"("Acquire"=w308, "Running"=w309, "ShutterOpen"=TRUE, "JYCCDLib.IJYCCDReqd"=w301) -> ("Raw Data"=w298:i32[][])  [unwired: 6 in, 1 out]
                                n146 = Index Array(array=w298, index (row)=0) -> (element=w297:i32[])  [unwired: 1 in]
                                n147 = local read "Wavelengths (nm)"() -> (w311:dbl[])
                                n148 = Increment(x=w316) -> (x+1=w302:i32)
                                n149 = Number To Decimal String(number=w302) -> (decimal integer string=w305:string)  [unwired: 1 in]
                                n150 = Concatenate Strings(w305, "/" ("string"), w306) -> (w304:string)
                                n151 = local write "CCD Current Rep."(w304) -> ()
                                n152 = Build Array (concatenate)(w297, w315) -> (w314:i32[][])
                                n153 = call "Symphony Average Spectra.vi"("Repetitions"=w302, "Raw Spectra"=w314) -> ("Raw Spectrum"=w313:dbl[])
                                n154 = local read "Start"() -> (w310:bool)
                                n155 = call "Spectrum Merge Wavelengths v10.5.0.vi"("Wavelengths (nm)"=w311, "Raw Spectrum"=w313) -> ("Spectrum-Cluster"=w312:T13)  [unwired: 1 out]
                                }
                                }
                                frame True {
                                # "simulate spectrum"
                                n156 = call "Mapping Simulated Spectrum v10.1.0.vi"() -> ("Simulated Spectrum"=w317:cluster{i32[], dbl[]}[])
                                }
                                }
                                n157 = local read "Target Position"() -> (w281:T8)
                                n158 = Index Array(array=w275, index=0 ("Index")) -> (element=w274:T14)
                                n159 = call "Mapping Merge Live Data v10.2.1.vi"("New Spectrum"=w274, "Target Position"=w281, "X in (1D)"=w289, "Y in (1D)"=w288, "L in (2D)"=w287, "I in (2D)"=w286, "Step Size"=w272) -> ("Live Data"=w280:dbl[][], "X out (1D)"=w283:dbl[], "Y out (1D)"=w282:dbl[], "L out (2D)"=w284:dbl[][], "I out (2D)"=w285:dbl[][])  [unwired: 4 in]
                                n160 = invoke class="VI Interface Type 0" method="Ctrl Val.Set"(reference=w291, "Control Name"="LiveData" ("Elementname"), "Value"=w280) -> ()  [unwired: 2 in, 5 out]
                                n161 = local write "Live Data"(w280) -> ()
                              }
                            }
                          }
                          frame #4 {
                            # "set new X"
                            n162 = Increment(x=w328) -> (x+1=w327:i32)
                            n163 = local read "Start"() -> (w321:bool)
                            n164 = Equal?(x=w326, y=w327) -> (x = y?=w318:bool)
                            n165 = Not(x=w321) -> (.not. x?=w320:bool)
                            n166 = Or(x=w318, y=w320) -> (x .or. y?=w319:bool)
                            n167 = case shown="False" w319 {
                              tunnel: w325 -> [w336 w344]
                              tunnel: [w335 w344] -> w322
                              tunnel: w324 -> [w334 _]
                              tunnel: w323 -> [w329 _]
                              frame False {
                                n168 = Unbundle By Name(w336) -> ("Drive X Set"=w337:dbl)
                                n169 = case shown="False" w334 {
                                tunnel: w337 -> [w340 w342]
                                tunnel: [w339 w343] -> w330
                                tunnel: w329 -> [w338 w341]
                                frame False {
                                n170 = Subtract(x=w340, y=w338) -> (x-y=w339:dbl)
                                }
                                frame True {
                                n171 = Add(x=w342, y=w341) -> (x+y=w343:dbl)
                                }
                                }
                                n172 = Divide(x=w330, y=w329) -> (x/y=w333:dbl)
                                n173 = Round To Nearest(number=w333) -> (nearest integer value=w332:dbl)
                                n174 = Multiply(x=w332, y=w329) -> (x*y=w331:dbl)
                                n175 = Bundle By Name(cluster=w336, "Drive X Set"=w331) -> (w335:T12)
                              }
                              frame True {
                              }
                            }
                            n176 = local write "Target Position"(w322) -> ()
                          }
                          frame #5 {
                            n177 = Tick Count (ms)() -> (millisecond timer value=w349:u32)
                            n178 = Subtract(x=w349, y=w348) -> (x-y=w351:u32)
                            n179 = Divide(x=w351, y=u32 1000) -> (x/y=w346:dbl)
                            n180 = Build Array (concatenate)(w347, w346) -> (w345:dbl[])
                          }
                        }
                        n181 = local read "Start"() -> (w201:bool)
                      }
                    }
                    frame #1 {
                      # "set new Y\nand move to new position"
                      n182 = Increment(x=w363) -> (x+1=w362:i32)
                      n183 = local read "Start"() -> (w353:bool)
                      n184 = Equal?(x=w361, y=w362) -> (x = y?=w355:bool)
                      n185 = local read "Simulate Drive"() -> (w356:bool)
                      n186 = Not(x=w353) -> (.not. x?=w354:bool)
                      n187 = Or(x=w355, y=w354) -> (x .or. y?=w352:bool)
                      n188 = case shown="False" w352 {
                        tunnel: w359 -> [w384 w385]
                        tunnel: [w383 w385] -> w357
                        tunnel: w360 -> [w378 _]
                        frame False {
                          n189 = Unbundle By Name(w384) -> ("Drive Y Set"=w382:dbl)
                          n190 = Add(x=w378, y=w382) -> (x+y=w379:dbl)
                          n191 = Divide(x=w379, y=w378) -> (x/y=w380:dbl)
                          n192 = Round To Nearest(number=w380) -> (nearest integer value=w381:dbl)
                          n193 = Multiply(x=w381, y=w378) -> (x*y=w377:dbl)
                          n194 = Bundle By Name(cluster=w384, "Drive Y Set"=w377) -> (w383:T12)
                        }
                        frame True {
                        }
                      }
                      n195 = case shown="False" w356 {
                        tunnel: w358 -> [w368 _]
                        tunnel: w357 -> [w367 _]
                        frame False {
                          n196 = local read "Current Position"() -> (w366:T4)
                          n197 = Unbundle By Name(w366) -> ("Voltages.Drive Y Voltage"=w365:dbl)
                          n198 = flat-sequence {
                            tunnel: w368 -> [w370]
                            tunnel: w367 -> [w371]
                            tunnel: w365 -> [w372]
                            tunnel: [w370] -> w369
                            tunnel: [w376] -> w364
                            tunnel: w369 -> [w375]
                            frame #0 {
                              n199 = control-ref of="Objective Running"() -> (w374:refnum<vi>)
                              n200 = call "ESA-C Move Axis To v10.5.2.vi"("Drive Connection Settings"=w370, "Axis"=2, "Current Voltage (V)"=w372, "Drive New Abs. Positions"=w371, "Running"=w374) -> ()  [unwired: 2 in]
                            }
                            frame #1 {
                              n201 = call "ESA-C Get Values.vi"("Drive Connection Settings"=w375) -> ("Drive Current Values"=w376:T4)
                            }
                          }
                          n202 = global write "Global Variables.vi" "Global Drive Position"(w364) -> ()
                          n203 = local write "Current Position"(w364) -> ()
                        }
                        frame True {
                        }
                      }
                      n204 = local write "Target Position"(w357) -> ()
                    }
                  }
                  n205 = local read "Start"() -> (w144:bool)
                }
              }
              frame #2 {
                # "conclude measurement"
                n206 = flat-sequence {
                  tunnel: w387 -> [w400]
                  tunnel: w386 -> [w399]
                  tunnel: w388 -> [w407]
                  frame #0 {
                    # "save data"
                    n207 = local read "Input Parameters"() -> (w393:T1)
                    n208 = global read "Global Variables.vi" "Global iHR Values"() -> (w396:T5)
                    n209 = global read "Global Variables.vi" "Global ITC Values"() -> (w397:T3)
                    n210 = local read "Spectra Params"() -> (w394:T6)
                    n211 = global read "Global Variables.vi" "Global CCD Temperature (C)"() -> (w395:dbl)
                    n212 = Unbundle By Name(w393) -> ("CCD Area"=w392:T7, "CCD Gain"=w390:u16, "CCD ADC"=w391:u16)
                    n213 = local read "Mapping Params"() -> (w389:T9)
                    n214 = call "Export_mappingFileName v10.5.1.vi"("ITC503 Current Values"=w397, "iHR Current Values"=w396, "Spectra Settings"=w394, "Mapping Parameters"=w389) -> ("Filename"=w403:string)  [unwired: 1 in]
                    "Filename" <- w403
                    n215 = local read "Live Data"() -> (w402:dbl[][])
                    n216 = Unbundle By Name(w389) -> ("Step Size"=w398:dbl)
                    n217 = call "Mapping Merge Real Positions v10.2.1.vi"("Live Data In"=w402, "X in (1D)"=w400, "Y in (1D)"=w399, "Step Size"=w398) -> ("Live Data Out"=w401:dbl[][])  [unwired: 11 in]
                    "Full Data" <- w401
                    n218 = call "Export_2DtoTxt v10.5.1.vi"("ITC503 Current Values"=w397, "iHR Current Values"=w396, "CCD Temperature"=w395, "CCD Area"=w392, "CCD ADC"=w391, "CCD Gain"=w390, "Export Type"="Mapping", "Spectra Settings"=w394, "Filename"=w403, "Data (2D)"=w401, "Mapping Parameters"=w389) -> ()  [unwired: 8 in, 1 out]
                  }
                  frame #1 {
                    # "reset indicators"
                    n219 = case shown="False" w407 {
                      frame False {
                      }
                      frame True {
                      }
                    }
                    n220 = local write "Start"(FALSE ("Start")) -> ()
                    n221 = local write "CCD Current Rep."("0/0" ("CCD3000 Current Rep.")) -> ()
                    n222 = global write "Global Variables.vi" "Mapping Running?"(FALSE ("Mapping Running?")) -> ()
                    n223 = property on="Measuring" class="Bool (strict)"("BoolText.Text"="" ("Boolescher Text.Text")) -> ()  [unwired: 2 in, 2 out]
                    n224 = property on="Measuring" class="Bool (strict)"("Blinking"=FALSE ("Measuring")) -> ()  [unwired: 2 in, 2 out]
                  }
                }
              }
            }
          }
        }
        n225 = local read "Exit"() -> (w41:bool)
      }
    }
    frame #2 {
      n226 = invoke class="VI Interface Type 0" method="Ctrl Val.Set"(reference=w412, "Control Name"="Exit" ("Elementname"), "Value"=TRUE) -> ()  [unwired: 2 in, 5 out]
      n227 = local read "AutoClose"() -> (w411:bool)
      n228 = flat-sequence {
        tunnel: w411 -> [w415]
        frame #0 {
          # "reset and close"
          n229 = control-ref of="Dieses VI"() -> (w418:refnum<vi>)
          n230 = global write "Global Variables.vi" "Mapping Open?"(FALSE ("Mapping Open?")) -> ()
          n231 = invoke class="VI" method="Default Vals.Reinit All"(reference=w418) -> (reference out=w416:refnum<vi>)  [unwired: 2 in, 2 out]
          n232 = property on="Measuring" class="Bool (strict)"("BoolText.Text"="" ("Boolescher Text.Text")) -> ()  [unwired: 2 in, 2 out]
          n233 = property class="App"() -> ("App.Kind"=w419:T15)  [unwired: 2 in, 2 out]
          n234 = case shown="\"Development System\"" w419 {
            tunnel: w416 -> [w421 w423]
            tunnel: w415 -> [_ w422]
            frame "invalid app kind", Default {
              n235 = invoke on="Invoke Node" class="VI" method="FP.Close"(reference=w421) -> ()  [unwired: 2 in, 3 out]
            }
            frame "Development System" {
              n236 = case shown="True" w422 {
                tunnel: w423 -> [_ w424]
                frame False {
                }
                frame True {
                  n237 = invoke on="Invoke Node" class="VI" method="FP.Close"(reference=w424) -> ()  [unwired: 2 in, 3 out]
                }
              }
            }
          }
        }
      }
    }
  }
